vi "get_leylines.vi"(10 "NotifierReff":T1, 11 "Waypoint queue":refnum<queue>) -> (1 "Other leyline":dbl, 2 "Final leyline":dbl, 3 "Waypoint queue out":refnum<queue>)   [LabVIEW 2013]
doc: "This VI takes the current+next waypoint, as well as the abs wind+irons range. The VI returns the two lines along which to tack, both offset by half of the irons range from the abs wind direction. The \"Final leyline\" is the one that ends up heading nearer the next waypoint.\n\nEric Schneider, September 2014"
uses:
  Classes/Waypoint/Waypoint.lvclass
  Data/TypeDefs/Notifiers.ctl
  Data/TypeDefs/UTM Location.ctl
  Data/TypeDefs/Sail Set Suggestions.ctl
  Data/TypeDefs/Rudder Set Suggestions.ctl
  Data/TypeDefs/OverrideInformation.ctl
  Data/TypeDefs/OverrideMode.ctl
  Data/TypeDefs/MotorSetup.ctl
  Data/TypeDefs/DynamixelSetupInfo.ctl
  Data/TypeDefs/AirmarStatus.ctl
  Data/TypeDefs/HardwareOnline.ctl
  Data/TypeDefs/DynamixelCycleTracker.ctl
  Data/TypeDefs/RC Input Values.ctl
  Utilities/Math/Angles/Angle/Angle.lvclass
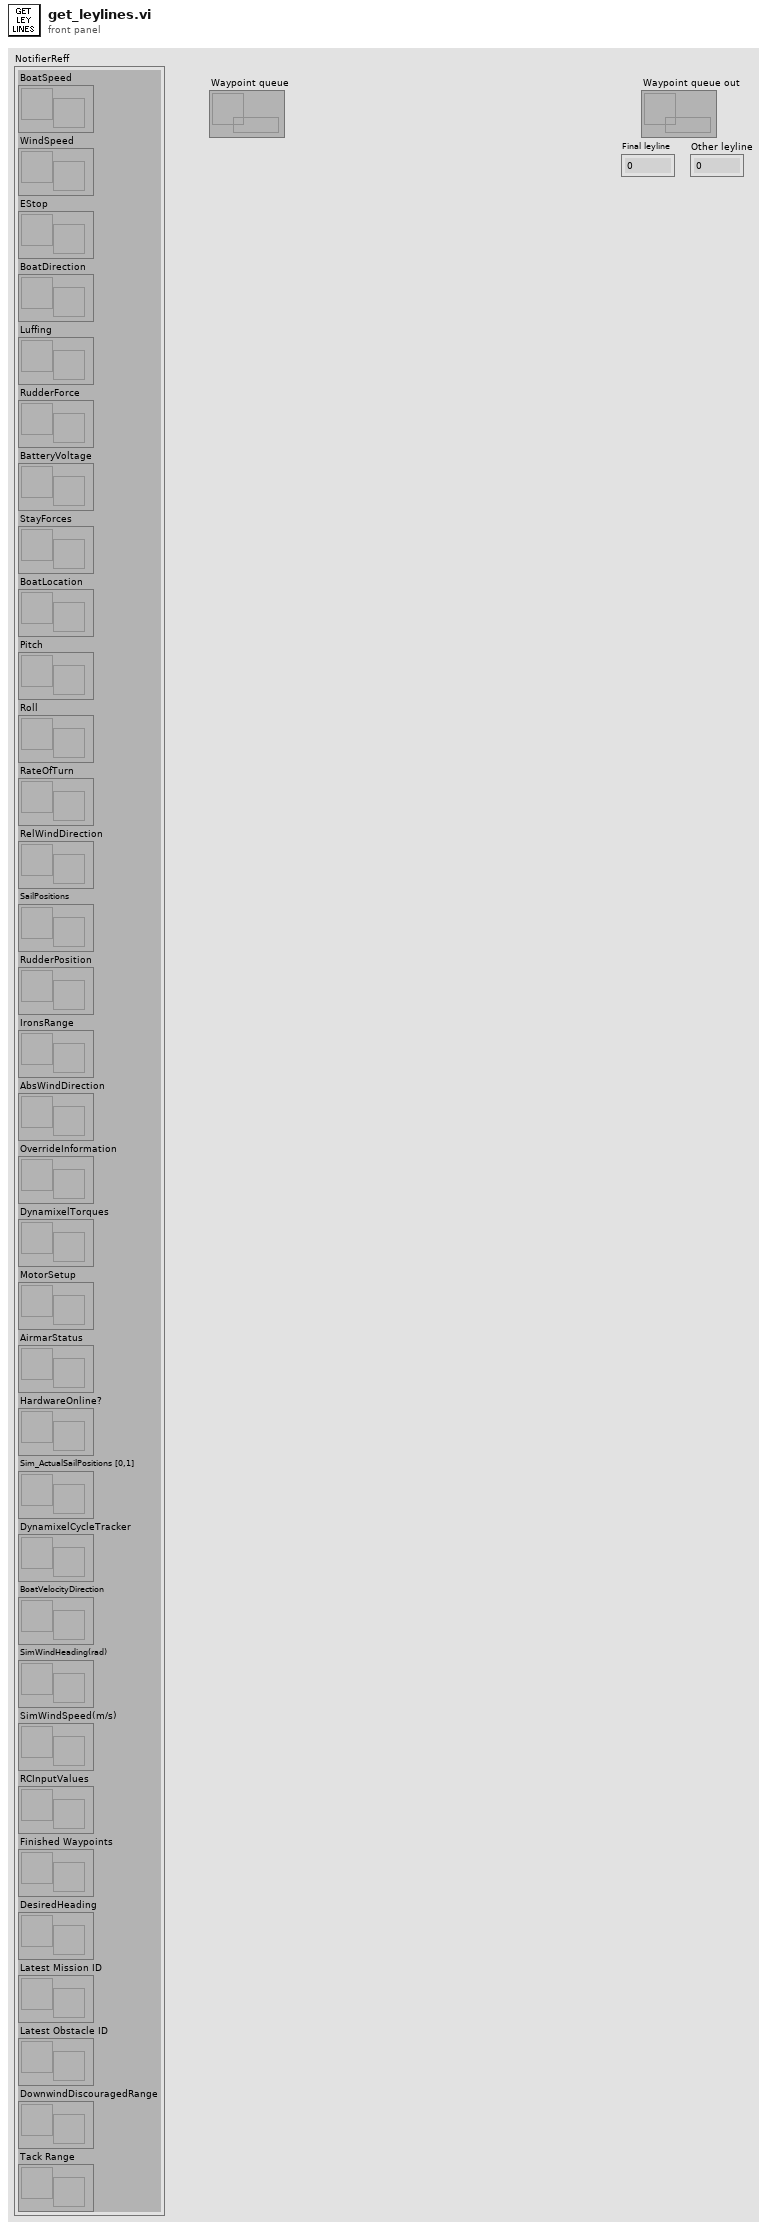
[diagram p1: front panel]
types:
  T1 = typedef "Notifiers.ctl" = cluster{"BoatSpeed":refnum<notifier>, "WindSpeed":refnum<notifier>, "EStop":refnum<notifier>, "BoatDirection":refnum<notifier>, "Luffing":refnum<notifier>, "RudderForce":refnum<notifier>, "BatteryVoltage":refnum<notifier>, "StayForces":refnum<notifier>, "BoatLocation":refnum<notifier>, "Pitch":refnum<notifier>, "Roll":refnum<notifier>, "RateOfTurn":refnum<notifier>, "RelWindDirection":refnum<notifier>, "SailPositions":refnum<notifier>, "RudderPosition":refnum<notifier>, "IronsRange":refnum<notifier>, "AbsWindDirection":refnum<notifier>, "OverrideInformation":refnum<notifier>, "DynamixelTorques":refnum<notifier>, "MotorSetup":refnum<notifier>, "AirmarStatus":refnum<notifier>, "HardwareOnline?":refnum<notifier>, "Sim_ActualSailPositions [0,1]":refnum<notifier>, "DynamixelCycleTracker":refnum<notifier>, "BoatVelocityDirection":refnum<notifier>, "SimWindHeading(rad)":refnum<notifier>, "SimWindSpeed(m/s)":refnum<notifier>, "RCInputValues":refnum<notifier>, "Finished Waypoints":refnum<notifier>, "DesiredHeading":refnum<notifier>, "Latest Mission ID":refnum<notifier>, "Latest Obstacle ID":refnum<notifier>, "DownwindDiscouragedRange":refnum<notifier>, "Tack Range":refnum<notifier>}
  T2 = typedef "UTM Location.ctl" = cluster{"UTM Zone":dbl, "Hemisphere":enum16{"North", "South"}, "East":dbl, "North":dbl}
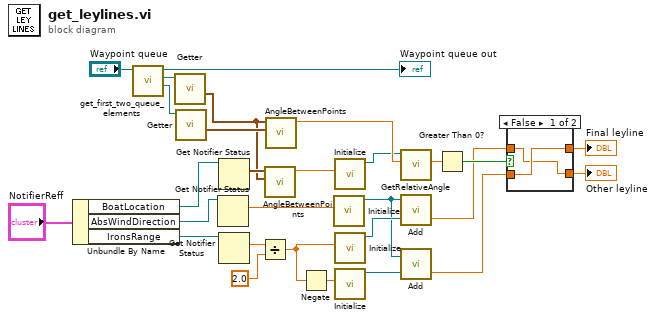
[diagram p0: block diagram]
diagram:
  n1 = Unbundle By Name("NotifierReff") -> ("BoatLocation"=w6:refnum<notifier>, "AbsWindDirection"=w22:refnum<notifier>, "IronsRange"=w23:refnum<notifier>)
  n2 = call "get_first_two_queue_elements.vi"("Waypoint queue"="Waypoint queue") -> ("Second element"=w28:refnum<class "Waypoint.lvclass">, "First element"=w26:refnum<class "Waypoint.lvclass">, "Waypoint queue out"=→"Waypoint queue out":refnum<queue>)  [unwired: 8 in]
  n3 = call "Getter.vi"("Waypoint In"=w26) -> ("Coords"=w1:T2)  [unwired: 6 in, 4 out]
  n4 = call "Getter.vi"("Waypoint In"=w28) -> ("Coords"=w3:T2)  [unwired: 6 in, 4 out]
  n5 = Get Notifier Status(notifier=w22) -> (current notification=w21:dbl)  [unwired: 1 in, 4 out]
  n6 = Get Notifier Status(notifier=w6) -> (current notification=w4:T2)  [unwired: 1 in, 4 out]
  n7 = Get Notifier Status(notifier=w23) -> (current notification=w9:dbl)  [unwired: 1 in, 4 out]
  n8 = Divide(x=w9, y=2.0) -> (x/y=w7:dbl)
  n9 = call "AngleBetweenPoints.vi"("Point 2"=w1, "Point 1"=w4) -> ("Angle from P1 to P2"=w5:dbl)  [unwired: 9 in]
  n10 = call "AngleBetweenPoints.vi"("Point 2"=w3, "Point 1"=w1) -> ("Angle from P1 to P2"=w16:dbl)  [unwired: 9 in]
  n11 = Negate(x=w7) -> (-x=w20:dbl)
  n12 = call "Initialize.vi"("Input Angle (Deg.)"=w21) -> ("Angle out"=w17:refnum<class "Angle.lvclass">)  [unwired: 9 in, 1 out]
  n13 = call "Initialize.vi"("Input Angle (Deg.)"=w5) -> ("Angle out"=w2:refnum<class "Angle.lvclass">)  [unwired: 9 in, 1 out]
  n14 = call "Initialize.vi"("Input Angle (Deg.)"=w7) -> ("Angle out"=w19:refnum<class "Angle.lvclass">)  [unwired: 9 in, 1 out]
  n15 = call "Initialize.vi"("Input Angle (Deg.)"=w20) -> ("Angle out"=w18:refnum<class "Angle.lvclass">)  [unwired: 9 in, 1 out]
  n16 = call "GetRelativeAngle.vi"("Boat Heading (Deg.)"=w16, "Angle in"=w2) -> ("Relative Angle FROM P2 TO P1 (deg)"=w15:dbl)  [unwired: 6 in, 3 out]
  n17 = call "Add.vi"("AngleAdd"=w19, "Angle in"=w17) -> ("Output"=w13:dbl)  [unwired: 1 out]
  n18 = call "Add.vi"("AngleAdd"=w18, "Angle in"=w17) -> ("Output"=w12:dbl)  [unwired: 1 out]
  n19 = Greater Than 0?(x=w15) -> (x > 0?=w14:bool)
  n20 = case shown="False" w14 {
    tunnel: w13 -> [w29 w31]
    tunnel: w12 -> [w30 w32]
    tunnel: [w29 w32] -> w10
    tunnel: [w30 w31] -> w11
    frame False {
    }
    frame True {
    }
  }
  "Final leyline" <- w11
  "Other leyline" <- w10
